vi "array -- bilinear regression 3D -- V2.vi"(7 "action":T3, 9 "fit map IN":map{T1, dbl}(c390), 11 "xywz IN":T2={"x"=[0.0, 0.0, 0.0, -1.0, -1.0, -1.0, 1.0, 1.0, 1.0], "y"=[-1.0, 0.0, 1.0, -1.0, 0.0, 1.0, -1.0, 0.0, 1.0], "z"=[1.0, 0.0, 1.0, 4.0, 1.0, 0.0, 0.0, 1.0, 4.0], "w"=[-1.0, 0.0, 1.0, -1.0, 0.0, 1.0, -1.0, 0.0, 1.0]}) -> (1 "fit map out":map{T1, dbl}(c390), 3 "xywz OUT":T2={"x"=[0.0, 0.0, 0.0, -1.0, -1.0, -1.0, 1.0, 1.0, 1.0], "y"=[-1.0, 0.0, 1.0, -1.0, 0.0, 1.0, -1.0, 0.0, 1.0], "z"=[1.0, 0.0, 1.0, 4.0, 1.0, 0.0, 0.0, 1.0, 4.0], "w"=[-1.0, 0.0, 1.0, -1.0, 0.0, 1.0, -1.0, 0.0, 1.0]})   [LabVIEW 2021]
uses:
  array -- fit control .ctl
  array -- bilinear regression 2D.ctl
  <vilib>/Analysis/baseanly.llb/Matrix Type of Inverse Matrix.ctl
  <vilib>/Analysis/baseanly.llb/Real A x B.vi
  <vilib>/Analysis/Matrix/Numeric/Conversions/Array To Matrix - RA2.vi
  <vilib>/Analysis/baseanly.llb/Real Inverse Matrix.vi
  <vilib>/Analysis/Matrix/Numeric/Conversions/Matrix To Array - RM.vi
  <vilib>/Analysis/NI_AALBase.lvlib
  <vilib>/Analysis/Matrix/NI_Matrix.lvlib
panel:
  out "w":dbl[](array[numeric])=[-1.0, 0.0, 1.0, -1.0, 0.0, 1.0, -1.0, 0.0, 1.0]
  out "y":dbl[](array[numeric])=[-1.0, 0.0, 1.0, -1.0, 0.0, 1.0, -1.0, 0.0, 1.0]
  out "fit  IN":dbl[](array[numeric])=[1.9, 2.6, 3.3, 1.0, 2.7, 3.9]
  out "fit OUT":dbl[](array[numeric])=[1.0, 1.0, 1.0, 0.0, 0.0, 0.0]
  out "z":dbl[](array[numeric])=[1.0, 0.0, 1.0, 4.0, 1.0, 0.0, 0.0, 1.0, 4.0]
  out "x":dbl[](array[numeric])=[0.0, 0.0, 0.0, -1.0, -1.0, -1.0, 1.0, 1.0, 1.0]
  # "s"
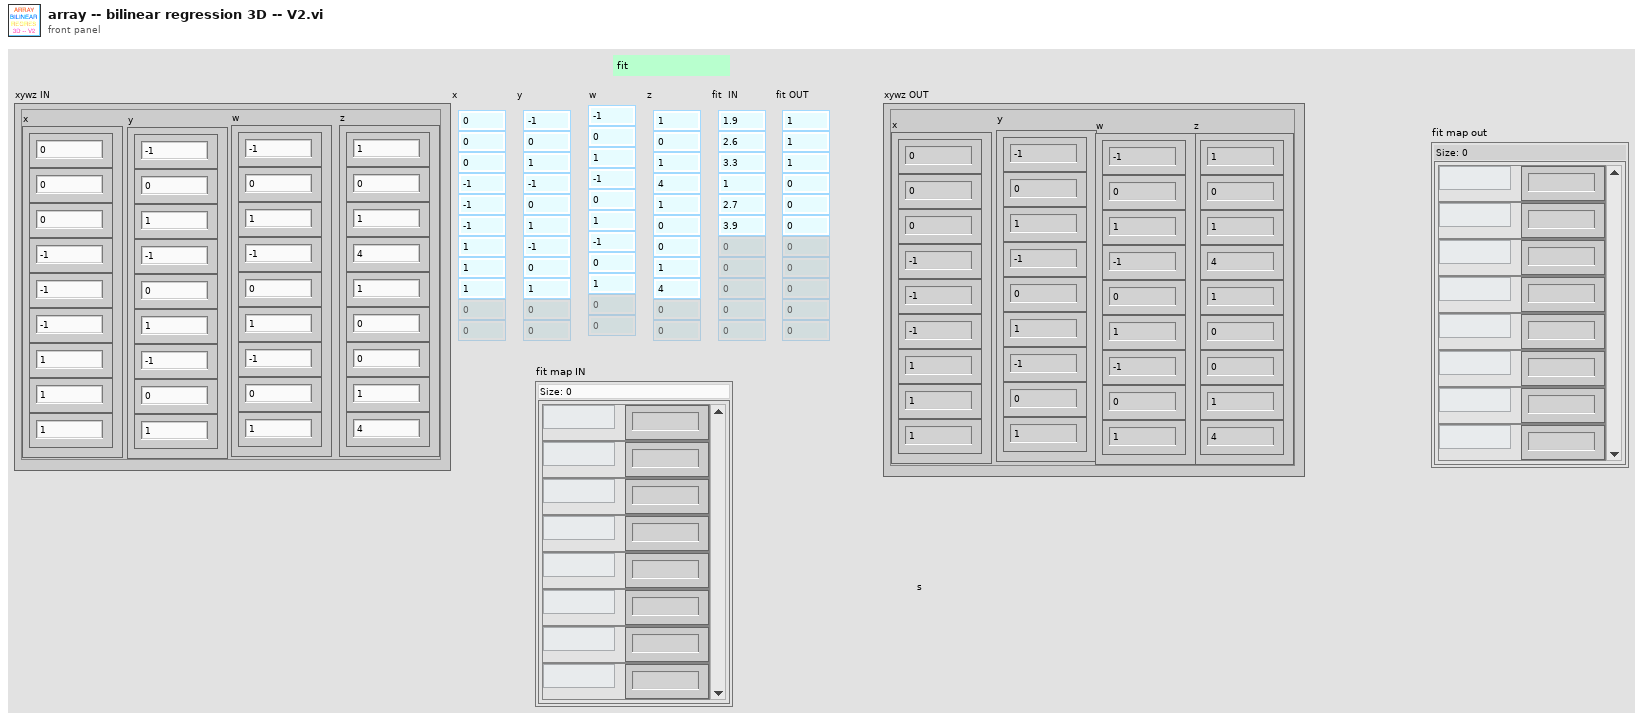
[diagram p1: front panel]
types:
  T1 = typedef "array -- bilinear regression 2D.ctl" = enum16{"1", "x", "y", "xx", "xy", "yy", "xxy", "xyy", "yyy", "xxx", "xxyy", "xyyy", "xxxy", "yyyy", "xxxx", "xxz", "xyz", "yyz", "xz", "yz", "z", "wwz", "ywz", "xwz", "xxxw", "xxyw", "xyyw", "yyyw", "xxww", "xyww", "yyww", "xwww", "ywww", "wwww", "ww", "xw", "yw", "w", "wz"}
  T2 = cluster{"x":dbl[], "y":dbl[], "z":dbl[], "w":dbl[]}
  T3 = typedef "array -- fit control .ctl" = enum16{"fit", "calc", "check", "init"}
  T4 = typedef "NI_AALBase.lvlib/Matrix Type of Inverse Matrix.ctl" = enum32{"General", "Positive Definite", "Lower Triangular", "Upper Triangular"}
  T5 = typedef "NI_Matrix.lvlib/RealMatrix.ctl" = dbl[][]
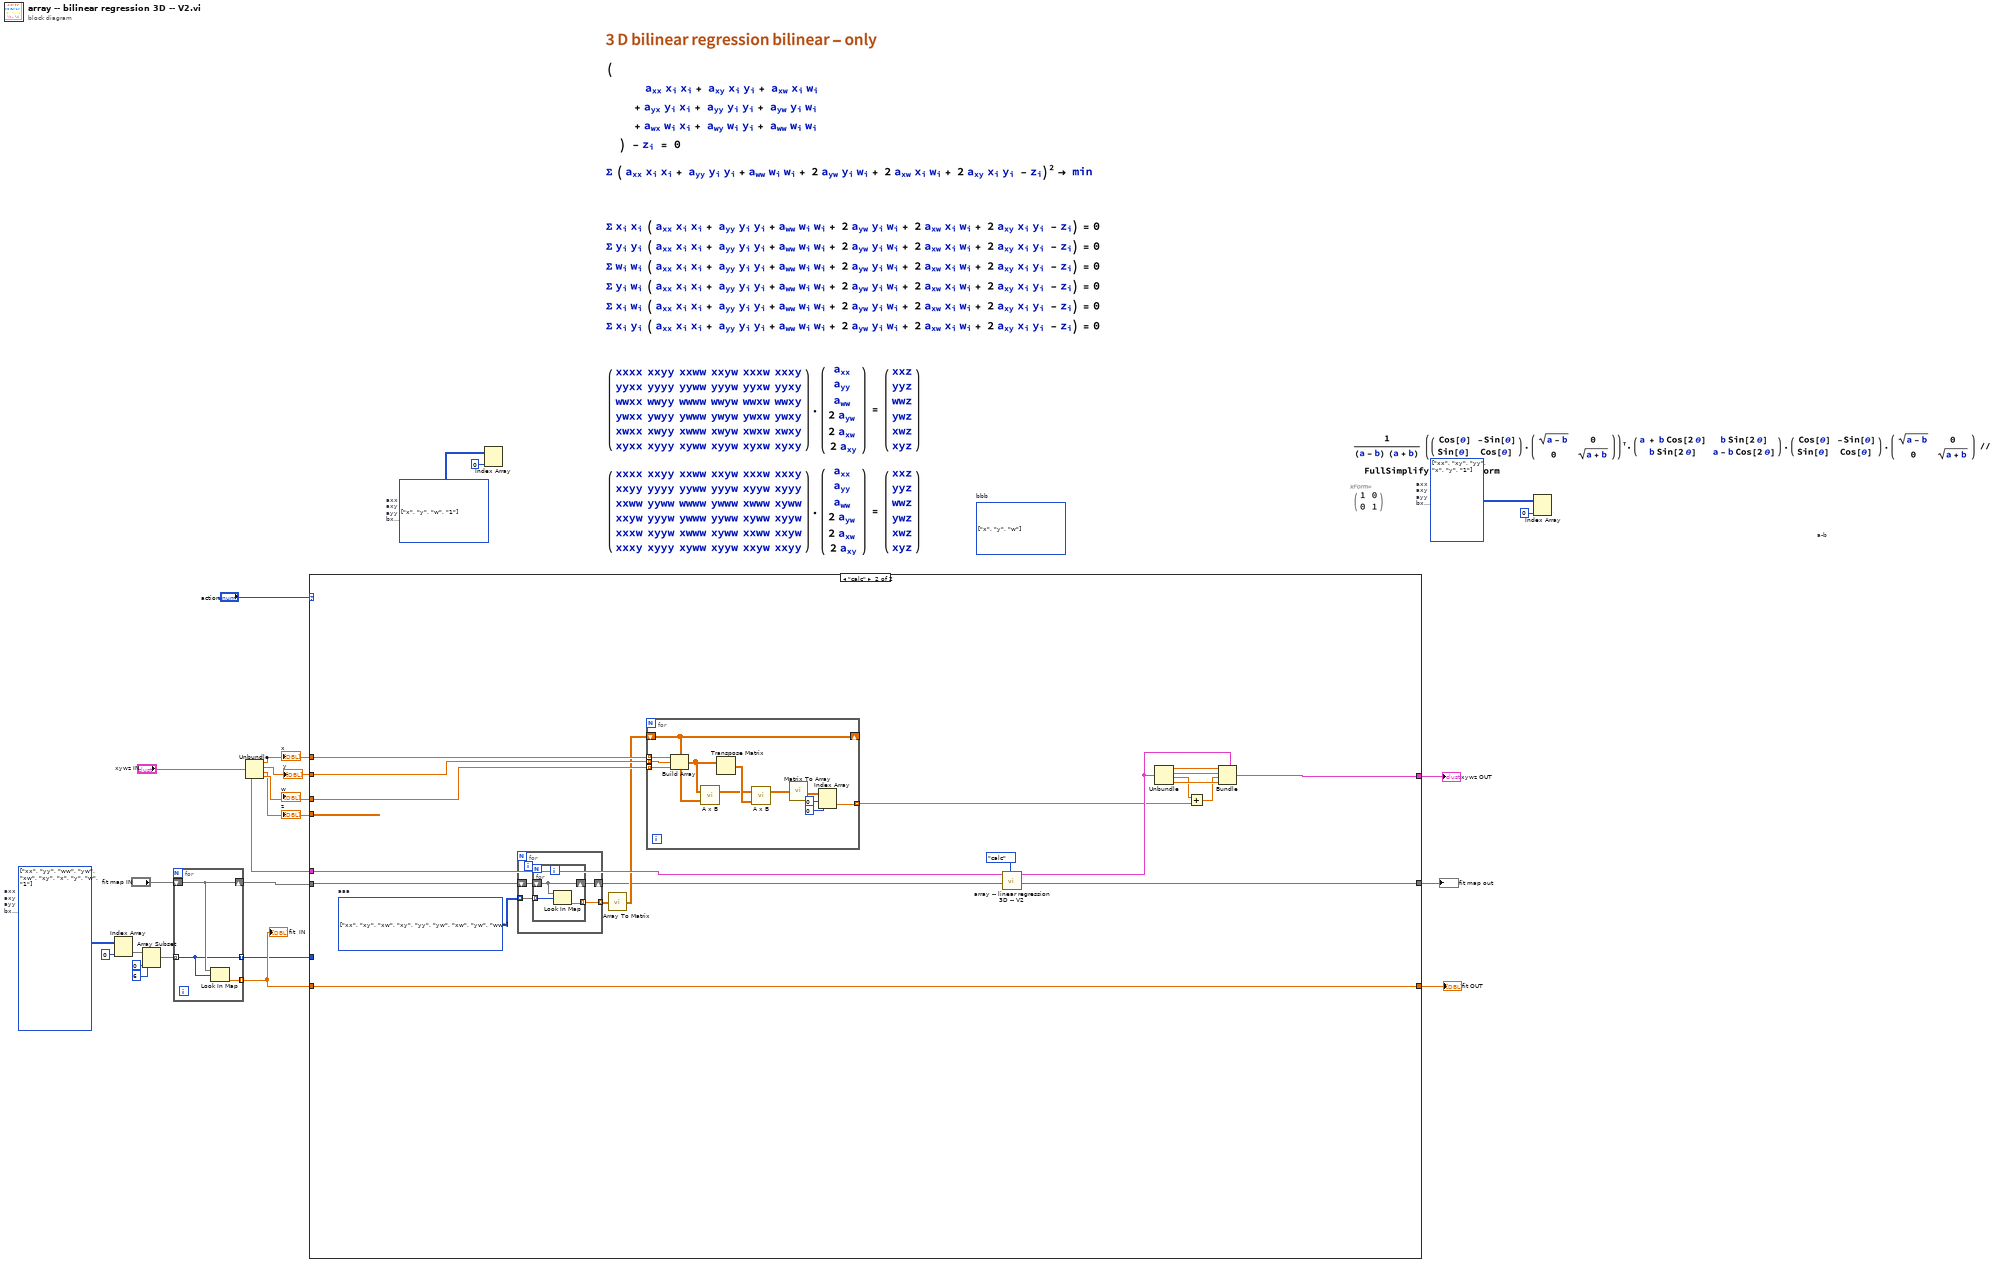
[diagram p0: block diagram]
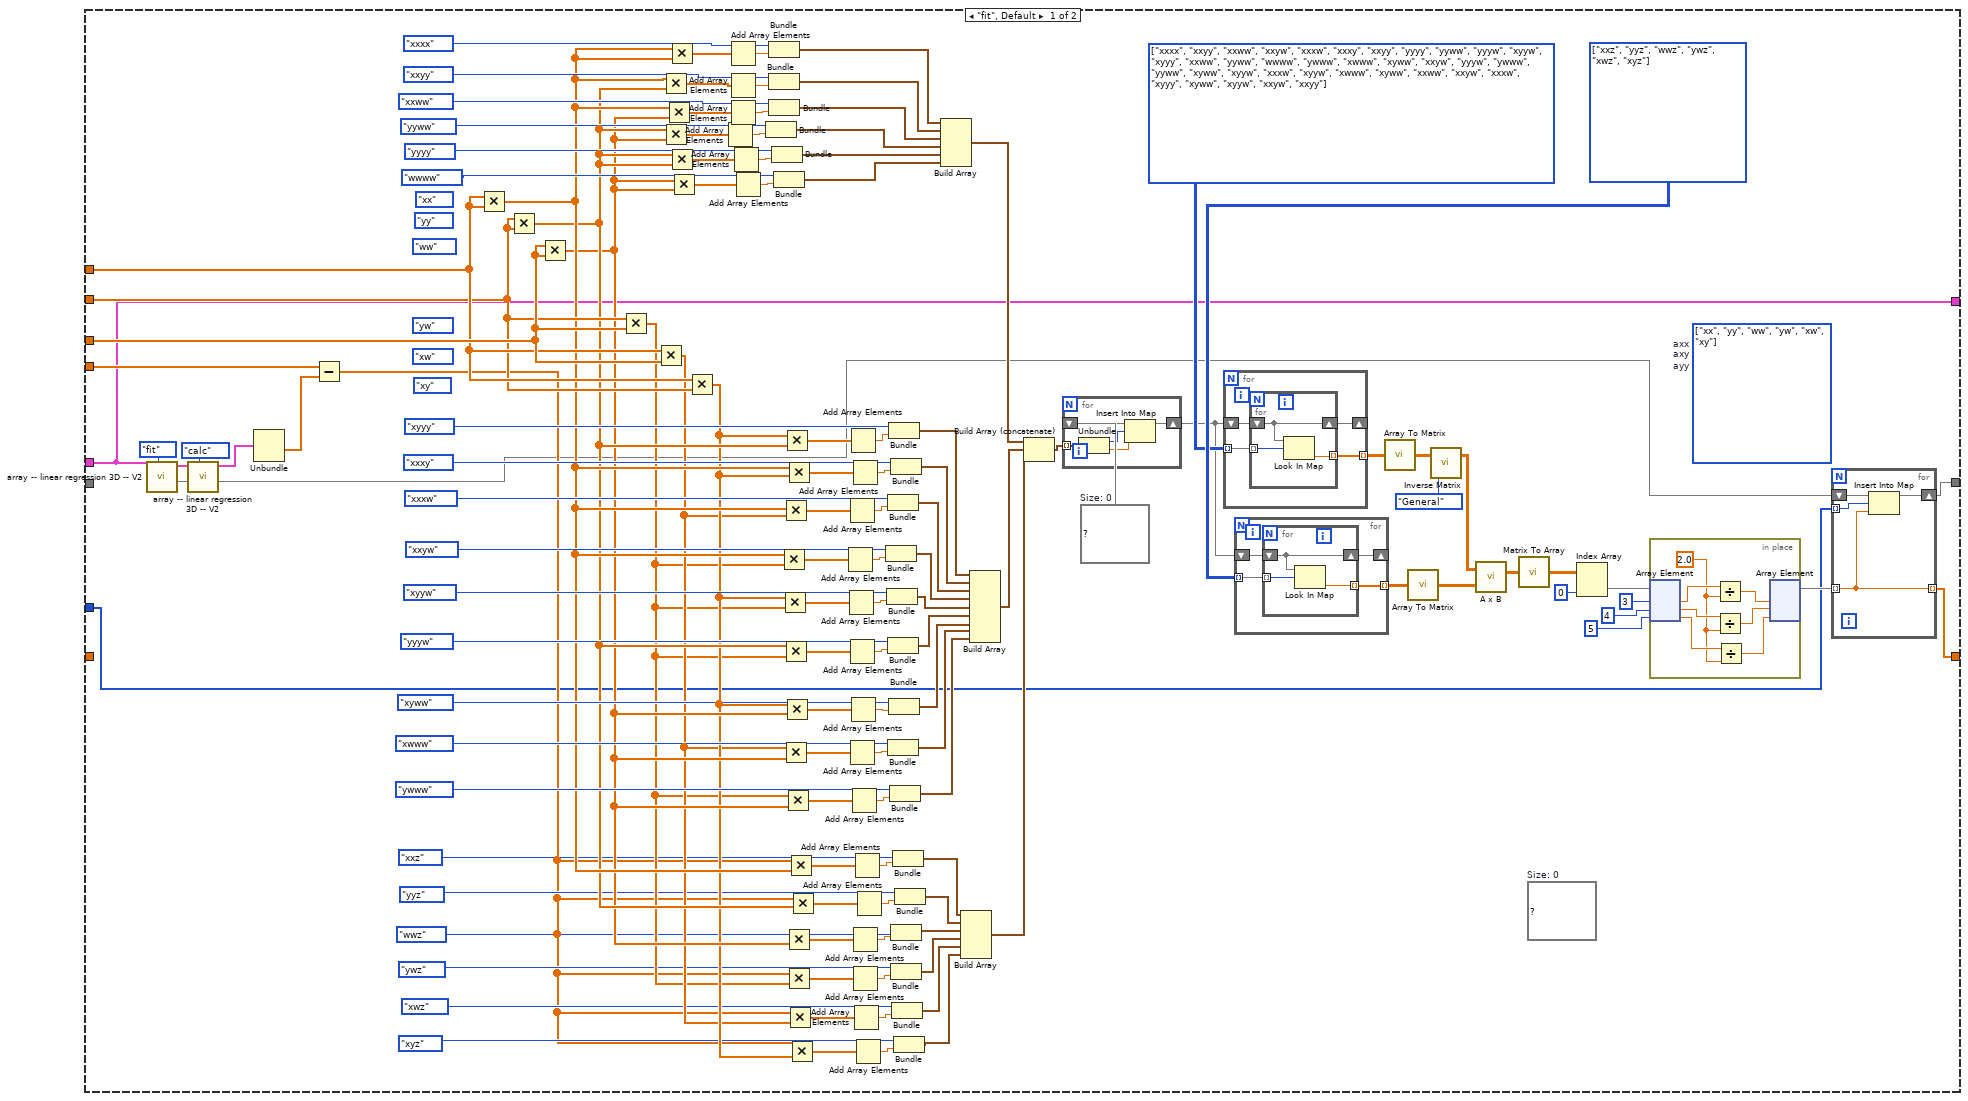
[diagram p2: hidden frame]
diagram:
  (unwired) T1[][] [[enum."x"], [enum."y"], [enum."w"]] items=["1", "x", "y", "xx", "xy", "yy", "xxy", "xyy", "yyy", "xxx", "xxyy", "xyyy", "xxxy", "yyyy", "xxxx", "xxz", "xyz", "yyz", "xz", "yz", "z", "wwz", "ywz", "xwz", "xxxw", "xxyw", "xyyw", "yyyw", "xxww", "xyww", "yyww", "xwww", "ywww", "wwww", "ww", "xw", "yw", "w", "wz"]  # bbb
  w15 = T1[][] [[enum."x"], [enum."y"], [enum."w"], [enum."1"]] items=["1", "x", "y", "xx", "xy", "yy", "xxy", "xyy", "yyy", "xxx", "xxyy", "xyyy", "xxxy", "yyyy", "xxxx", "xxz", "xyz", "yyz", "xz", "yz", "z", "wwz", "ywz", "xwz", "xxxw", "xxyw", "xyyw", "yyyw", "xxww", "xyww", "yyww", "xwww", "ywww", "wwww", "ww", "xw", "yw", "w", "wz"]  # axx axy ayy bx by c
  w17 = T1[][] [[enum."xx"], [enum."yy"], [enum."ww"], [enum."yw"], [enum."xw"], [enum."xy"], [enum."x"], [enum."y"], [enum."w"], [enum."1"]] items=["1", "x", "y", "xx", "xy", "yy", "xxy", "xyy", "yyy", "xxx", "xxyy", "xyyy", "xxxy", "yyyy", "xxxx", "xxz", "xyz", "yyz", "xz", "yz", "z", "wwz", "ywz", "xwz", "xxxw", "xxyw", "xyyw", "yyyw", "xxww", "xyww", "yyww", "xwww", "ywww", "wwww", "ww", "xw", "yw", "w", "wz"]  # axx axy ayy bx by c
  w19 = T1[][] [[enum."xx"], [enum."xy"], [enum."yy"], [enum."x"], [enum."y"], [enum."1"]] items=["1", "x", "y", "xx", "xy", "yy", "xxy", "xyy", "yyy", "xxx", "xxyy", "xyyy", "xxxy", "yyyy", "xxxx", "xxz", "xyz", "yyz", "xz", "yz", "z", "wwz", "ywz", "xwz", "xxxw", "xxyw", "xyyw", "yyyw", "xxww", "xyww", "yyww", "xwww", "ywww", "wwww", "ww", "xw", "yw", "w", "wz"]  # axx axy ayy bx by c
  # "a-b"
  n1 = Index Array(array=w17, index (col)=0 ("disabled index (col)")) -> (element=w12:T1[])  [unwired: 1 in]
  n2 = Array Subset(array=w12, index=0, length=6) -> (w3:T1[])
  n3 = for {
    shift-right: [w25] -> w2
    shift-left: "fit map IN" -> [w25]
    tunnel: w3 -> [w24] mode=indexing
    tunnel: [w26] -> w4 mode=indexing
    tunnel: [w24] -> w1 mode=indexing
    n4 = Look In Map(map=w25, key=w24) -> (value=w26:dbl)  [unwired: 1 in, 1 out]
  }
  "fit  IN" <- w4
  n5 = Unbundle("xywz IN") -> ("x"=w22:dbl[], "y"=w21:dbl[], "z"=w6:dbl[], "w"=w13:dbl[])
  "x" <- w22
  "z" <- w6
  "y" <- w21
  "w" <- w13
  n6 = case shown="\"calc\"" "action" {
    tunnel: w6 -> [w38 _]
    tunnel: w22 -> [w111 w200]
    tunnel: [w27 w187] -> w20
    tunnel: w21 -> [w110 w199]
    tunnel: w13 -> [w112 w198]
    tunnel: w2 -> [_ w188]
    tunnel: "xywz IN" -> [w31 w203]
    tunnel: [w31 w189] -> w9
    tunnel: [w40 w185] -> w8
    tunnel: w4 -> [_ w187]
    tunnel: w1 -> [w29 _]
    frame "fit", Default {
      (unwired) T1[][] [[enum."xx"], [enum."yy"], [enum."ww"], [enum."yw"], [enum."xw"], [enum."xy"]] items=["1", "x", "y", "xx", "xy", "yy", "xxy", "xyy", "yyy", "xxx", "xxyy", "xyyy", "xxxy", "yyyy", "xxxx", "xxz", "xyz", "yyz", "xz", "yz", "z", "wwz", "ywz", "xwz", "xxxw", "xxyw", "xyyw", "yyyw", "xxww", "xyww", "yyww", "xwww", "ywww", "wwww", "ww", "xw", "yw", "w", "wz"]  # axx axy ayy
      (unwired) map{T1, dbl} {}  # Size: 0
      w131 = T1[][] [[enum."xxz"], [enum."yyz"], [enum."wwz"], [enum."ywz"], [enum."xwz"], [enum."xyz"]] items=["1", "x", "y", "xx", "xy", "yy", "xxy", "xyy", "yyy", "xxx", "xxyy", "xyyy", "xxxy", "yyyy", "xxxx", "xxz", "xyz", "yyz", "xz", "yz", "z", "wwz", "ywz", "xwz", "xxxw", "xxyw", "xyyw", "yyyw", "xxww", "xyww", "yyww", "xwww", "ywww", "wwww", "ww", "xw", "yw", "w", "wz"]
      w130 = T1[][] [[enum."xxxx", enum."xxyy", enum."xxww", enum."xxyw", enum."xxxw", enum."xxxy"], [enum."xxyy", enum."yyyy", enum."yyww", enum."yyyw", enum."xyyw", enum."xyyy"], [enum."xxww", enum."yyww", enum."wwww", enum."ywww", enum."xwww", enum."xyww"], [enum."xxyw", enum."yyyw", enum."ywww", enum."yyww", enum."xyww", enum."xyyw"], [enum."xxxw", enum."xyyw", enum."xwww", enum."xyww", enum."xxww", enum."xxyw"], [enum."xxxw", enum."xyyy", enum."xyww", enum."xyyw", enum."xxyw", enum."xxyy"]] items=["1", "x", "y", "xx", "xy", "yy", "xxy", "xyy", "yyy", "xxx", "xxyy", "xyyy", "xxxy", "yyyy", "xxxx", "xxz", "xyz", "yyz", "xz", "yz", "z", "wwz", "ywz", "xwz", "xxxw", "xxyw", "xyyw", "yyyw", "xxww", "xyww", "yyww", "xwww", "ywww", "wwww", "ww", "xw", "yw", "w", "wz"]
      w133 = map{T1, dbl} {}  # Size: 0
      (unwired) array_--_bilinear_regression_2D."xy"
      (unwired) array_--_bilinear_regression_2D."xw"
      (unwired) array_--_bilinear_regression_2D."yw"
      (unwired) array_--_bilinear_regression_2D."ww"
      (unwired) array_--_bilinear_regression_2D."yy"
      (unwired) array_--_bilinear_regression_2D."xx"
      n7 = call "array -- linear regression 3D -- V2.vi"("action"=array_--_fit_control_."fit", "xyzw IN"=w31) -> ("fit map out"=w36:map{T1, dbl}, "xyz OUT"=w35:T2)  [unwired: 8 in]
      n8 = call "array -- linear regression 3D -- V2.vi"("action"=array_--_fit_control_."calc", "fit map IN"=w36, "xyzw IN"=w35) -> ("fit map out"=w32:map{T1, dbl}, "xyz OUT"=w37:T2)  [unwired: 7 in]
      n9 = Unbundle(w37) -> ("z"=w30:dbl[])  [unwired: 3 out]
      n10 = Subtract(x=w38, y=w30) -> (x-y=w39:dbl[])
      n11 = Multiply(x=w111, y=w111) -> (x*y=w55:dbl[])
      n12 = Multiply(x=w110, y=w110) -> (x*y=w54:dbl[])
      n13 = Multiply(x=w112, y=w112) -> (x*y=w53:dbl[])
      n14 = Multiply(x=w110, y=w112) -> (x*y=w50:dbl[])
      n15 = Multiply(x=w111, y=w112) -> (x*y=w51:dbl[])
      n16 = Multiply(x=w55, y=w54) -> (x*y=w126:dbl[])
      n17 = Multiply(x=w54, y=w53) -> (x*y=w123:dbl[])
      n18 = Multiply(x=w55, y=w53) -> (x*y=w125:dbl[])
      n19 = Multiply(x=w55, y=w55) -> (x*y=w149:dbl[])
      n20 = Multiply(x=w54, y=w54) -> (x*y=w121:dbl[])
      n21 = Multiply(x=w53, y=w53) -> (x*y=w119:dbl[])
      n22 = Multiply(x=w111, y=w110) -> (x*y=w52:dbl[])
      n23 = Add Array Elements(numeric array=w123) -> (sum=w124:dbl)
      n24 = Add Array Elements(numeric array=w149) -> (sum=w148:dbl)
      n25 = Add Array Elements(numeric array=w126) -> (sum=w146:dbl)
      n26 = Add Array Elements(numeric array=w125) -> (sum=w143:dbl)
      n27 = Add Array Elements(numeric array=w121) -> (sum=w122:dbl)
      n28 = Add Array Elements(numeric array=w119) -> (sum=w120:dbl)
      n29 = Bundle(array_--_bilinear_regression_2D."yyww", "Numeric"=w124) -> (w118:cluster{T1, "Numeric":dbl})  [unwired: 1 in]
      n30 = Bundle(array_--_bilinear_regression_2D."xxxx", "Numeric"=w148) -> (w127:cluster{T1, "Numeric":dbl})  [unwired: 1 in]
      n31 = Bundle(array_--_bilinear_regression_2D."xxyy", "Numeric"=w146) -> (w128:cluster{T1, "Numeric":dbl})  [unwired: 1 in]
      n32 = Bundle(array_--_bilinear_regression_2D."xxww", "Numeric"=w143) -> (w129:cluster{T1, "Numeric":dbl})  [unwired: 1 in]
      n33 = Bundle(array_--_bilinear_regression_2D."yyyy", "Numeric"=w122) -> (w114:cluster{T1, "Numeric":dbl})  [unwired: 1 in]
      n34 = Bundle(array_--_bilinear_regression_2D."wwww", "Numeric"=w120) -> (w113:cluster{T1, "Numeric":dbl})  [unwired: 1 in]
      n35 = Multiply(x=w55, y=w50) -> (x*y=w104:dbl[])
      n36 = Multiply(x=w52, y=w50) -> (x*y=w102:dbl[])
      n37 = Multiply(x=w55, y=w51) -> (x*y=w106:dbl[])
      n38 = Multiply(x=w54, y=w50) -> (x*y=w100:dbl[])
      n39 = Multiply(x=w51, y=w53) -> (x*y=w96:dbl[])
      n40 = Multiply(x=w52, y=w54) -> (x*y=w154:dbl[])
      n41 = Multiply(x=w52, y=w53) -> (x*y=w98:dbl[])
      n42 = Multiply(x=w50, y=w53) -> (x*y=w94:dbl[])
      n43 = Multiply(x=w55, y=w52) -> (x*y=w108:dbl[])
      n44 = Multiply(x=w39, y=w53) -> (x*y=w66:dbl[])
      n45 = Multiply(x=w39, y=w50) -> (x*y=w68:dbl[])
      n46 = Multiply(x=w39, y=w51) -> (x*y=w70:dbl[])
      n47 = Multiply(x=w39, y=w55) -> (x*y=w62:dbl[])
      n48 = Multiply(x=w39, y=w52) -> (x*y=w72:dbl[])
      n49 = Multiply(x=w39, y=w54) -> (x*y=w64:dbl[])
      n50 = Add Array Elements(numeric array=w104) -> (sum=w105:dbl)
      n51 = Add Array Elements(numeric array=w102) -> (sum=w103:dbl)
      n52 = Add Array Elements(numeric array=w106) -> (sum=w107:dbl)
      n53 = Add Array Elements(numeric array=w100) -> (sum=w101:dbl)
      n54 = Add Array Elements(numeric array=w96) -> (sum=w97:dbl)
      n55 = Add Array Elements(numeric array=w154) -> (sum=w141:dbl)
      n56 = Add Array Elements(numeric array=w98) -> (sum=w99:dbl)
      n57 = Add Array Elements(numeric array=w94) -> (sum=w95:dbl)
      n58 = Add Array Elements(numeric array=w108) -> (sum=w109:dbl)
      n59 = Add Array Elements(numeric array=w66) -> (sum=w67:dbl)
      n60 = Add Array Elements(numeric array=w68) -> (sum=w69:dbl)
      n61 = Add Array Elements(numeric array=w70) -> (sum=w71:dbl)
      n62 = Add Array Elements(numeric array=w62) -> (sum=w63:dbl)
      n63 = Add Array Elements(numeric array=w72) -> (sum=w73:dbl)
      n64 = Add Array Elements(numeric array=w64) -> (sum=w65:dbl)
      n65 = Bundle(array_--_bilinear_regression_2D."xxyw", "Numeric"=w105) -> (w79:cluster{T1, "Numeric":dbl})  [unwired: 1 in]
      n66 = Bundle(array_--_bilinear_regression_2D."xyyw", "Numeric"=w103) -> (w78:cluster{T1, "Numeric":dbl})  [unwired: 1 in]
      n67 = Bundle(array_--_bilinear_regression_2D."xxxw", "Numeric"=w107) -> (w80:cluster{T1, "Numeric":dbl})  [unwired: 1 in]
      n68 = Bundle(array_--_bilinear_regression_2D."yyyw", "Numeric"=w101) -> (w77:cluster{T1, "Numeric":dbl})  [unwired: 1 in]
      n69 = Bundle(array_--_bilinear_regression_2D."xwww", "Numeric"=w97) -> (w75:cluster{T1, "Numeric":dbl})  [unwired: 1 in]
      n70 = Bundle(array_--_bilinear_regression_2D."xyyy", "Numeric"=w141) -> (w82:cluster{T1, "Numeric":dbl})  [unwired: 1 in]
      n71 = Bundle(array_--_bilinear_regression_2D."xyww", "Numeric"=w99) -> (w76:cluster{T1, "Numeric":dbl})  [unwired: 1 in]
      n72 = Bundle(array_--_bilinear_regression_2D."ywww", "Numeric"=w95) -> (w74:cluster{T1, "Numeric":dbl})  [unwired: 1 in]
      n73 = Bundle(array_--_bilinear_regression_2D."xxxy", "Numeric"=w109) -> (w81:cluster{T1, "Numeric":dbl})  [unwired: 1 in]
      n74 = Bundle(array_--_bilinear_regression_2D."wwz", "Numeric"=w67) -> (w59:cluster{T1, "Numeric":dbl})  [unwired: 1 in]
      n75 = Bundle(array_--_bilinear_regression_2D."ywz", "Numeric"=w69) -> (w58:cluster{T1, "Numeric":dbl})  [unwired: 1 in]
      n76 = Bundle(array_--_bilinear_regression_2D."xwz", "Numeric"=w71) -> (w57:cluster{T1, "Numeric":dbl})  [unwired: 1 in]
      n77 = Bundle(array_--_bilinear_regression_2D."xxz", "Numeric"=w63) -> (w61:cluster{T1, "Numeric":dbl})  [unwired: 1 in]
      n78 = Bundle(array_--_bilinear_regression_2D."xyz", "Numeric"=w73) -> (w56:cluster{T1, "Numeric":dbl})  [unwired: 1 in]
      n79 = Bundle(array_--_bilinear_regression_2D."yyz", "Numeric"=w65) -> (w60:cluster{T1, "Numeric":dbl})  [unwired: 1 in]
      n80 = Build Array(w127, w128, w129, w118, w114, w113) -> (w84:cluster{T1, "Numeric":dbl}[])
      n81 = Build Array(w61, w60, w59, w58, w57, w56) -> (w43:cluster{T1, "Numeric":dbl}[])
      n82 = Build Array(w82, w81, w80, w79, w78, w77, w76, w75, w74) -> (w83:cluster{T1, "Numeric":dbl}[])
      n83 = Build Array (concatenate)(w84, w83, w43) -> (w85:cluster{T1, "Numeric":dbl}[])
      n84 = for {
        tunnel: w85 -> [w175] mode=indexing
        shift-right: [w176] -> w28
        shift-left: w133 -> [w177]
        n85 = Unbundle(w175) -> (w174:T1, "Numeric"=w173:dbl)
        n86 = Insert Into Map(map in=w177, key=w174, value=w173) -> (map out=w176:map{T1, dbl})  [unwired: 2 out]
      }
      n87 = for {
        tunnel: w130 -> [w181] mode=indexing
        shift-right: [w179] -> _
        shift-left: w28 -> [w180]
        tunnel: [w178] -> w139 mode=indexing
        n88 = for {
          tunnel: w181 -> [w183] mode=indexing
          shift-right: [w184] -> w179
          shift-left: w180 -> [w184]
          tunnel: [w182] -> w178 mode=indexing
          n89 = Look In Map(map=w184, key=w183) -> (value=w182:dbl)  [unwired: 1 in, 1 out]
        }
      }
      n90 = for {
        shift-right: [w168] -> _
        shift-left: w28 -> [w169]
        tunnel: w131 -> [w167] mode=indexing
        tunnel: [w166] -> w138 mode=indexing
        n91 = for {
          shift-right: [w172] -> w168
          shift-left: w169 -> [w172]
          tunnel: w167 -> [w171] mode=indexing
          tunnel: [w170] -> w166 mode=indexing
          n92 = Look In Map(map=w172, key=w171) -> (value=w170:dbl)  [unwired: 1 in, 1 out]
        }
      }
      n93 = call-poly <vilib>:"Array To Matrix.vi"("Real 2D Array"=w139) -> ("Real Matrix"=w134:T5)
      n94 = call-poly <vilib>:"Array To Matrix.vi"("Real 2D Array"=w138) -> ("Real Matrix"=w137:T5)
      n95 = call-poly <vilib>:"Inverse Matrix.vi"("matrix type"=Matrix_Type_of_Inverse_Matrix."General", "Input Matrix"=w134) -> ("Inverse Matrix"=w153:T5)  [unwired: 1 out]
      n96 = call-poly <vilib>:"A x B.vi"("B"=w137, "A"=w153) -> ("A x B"=w152:T5)  [unwired: 1 out]
      n97 = call-poly <vilib>:"Matrix To Array.vi"("Real Matrix"=w152) -> ("Real 2D Array"=w151:dbl[][])
      n98 = Index Array(array=w151, index (col)=0 ("disabled index (col)")) -> (element=w136:dbl[])  [unwired: 1 in]
      n99 = in-place {
        w159 = 2.0 ("y")
        n100 = in-place-array #1(w136, 3, 4, 5) -> (w165:dbl, w163:dbl, w161:dbl)
        n101 = Divide(x=w165, y=w159) -> (x/y=w164:dbl)
        n102 = Divide(x=w163, y=w159) -> (x/y=w162:dbl)
        n103 = Divide(x=w161, y=w159) -> (x/y=w160:dbl)
        n104 = in-place-array #1(w164, w162, w160) -> (w132:dbl[])  [unwired: 3 out]
      }
      n105 = for {
        shift-right: [w157] -> w40
        shift-left: w32 -> [w158]
        tunnel: w29 -> [w156] mode=indexing
        tunnel: w132 -> [w155] mode=indexing
        tunnel: [w155] -> w27 mode=indexing
        n106 = Insert Into Map(map in=w158, key=w156, value=w155) -> (map out=w157:map{T1, dbl})  [unwired: 2 out]
      }
    }
    frame "calc" {
      w201 = T1[][] [[enum."xx", enum."xy", enum."xw"], [enum."xy", enum."yy", enum."yw"], [enum."xw", enum."yw", enum."ww"]] items=["1", "x", "y", "xx", "xy", "yy", "xxy", "xyy", "yyy", "xxx", "xxyy", "xyyy", "xxxy", "yyyy", "xxxx", "xxz", "xyz", "yyz", "xz", "yz", "z", "wwz", "ywz", "xwz", "xxxw", "xxyw", "xyyw", "yyyw", "xxww", "xyww", "yyww", "xwww", "ywww", "wwww", "ww", "xw", "yw", "w", "wz"]  # aaa
      n107 = for {
        tunnel: w201 -> [w220] mode=indexing
        shift-right: [w218] -> w186
        shift-left: w188 -> [w219]
        tunnel: [w217] -> w202 mode=indexing
        n108 = for {
          tunnel: w220 -> [w222] mode=indexing
          shift-right: [w223] -> w218
          shift-left: w219 -> [w223]
          tunnel: [w221] -> w217 mode=indexing
          n109 = Look In Map(map=w223, key=w222) -> (value=w221:dbl)  [unwired: 1 in, 1 out]
        }
      }
      n110 = call-poly <vilib>:"Array To Matrix.vi"("Real 2D Array"=w202) -> ("Real Matrix"=w197:T5)
      n111 = for {
        tunnel: w200 -> [w215] mode=indexing
        tunnel: w199 -> [w214] mode=indexing
        tunnel: w198 -> [w213] mode=indexing
        shift-right: [w212] -> _
        shift-left: w197 -> [w212]
        tunnel: [w205] -> w190 mode=indexing
        n112 = Build Array(w215, w214, w213) -> (w211:T5)
        n113 = call-poly <vilib>:"A x B.vi"("B"=w212, "A"=w211) -> ("A x B"=w209:T5)  [unwired: 1 out]
        n114 = Transpose Matrix(1:w211) -> (0:w210:T5)
        n115 = call-poly <vilib>:"A x B.vi"("B"=w210, "A"=w209) -> ("A x B"=w216:T5)  [unwired: 1 out]
        n116 = call-poly <vilib>:"Matrix To Array.vi"("Real Matrix"=w216) -> ("Real 2D Array"=w208:dbl[][])
        n117 = Index Array(array=w208, index (row)=0, index (col)=0 ("disabled index (col)")) -> (element=w205:dbl)
      }
      n118 = call "array -- linear regression 3D -- V2.vi"("action"=array_--_fit_control_."calc", "fit map IN"=w186, "xyzw IN"=w203) -> ("fit map out"=w185:map{T1, dbl}, "xyz OUT"=w196:T2)  [unwired: 7 in]
      n119 = Unbundle(w196) -> ("x"=w195:dbl[], "y"=w194:dbl[], "z"=w192:dbl[], "w"=w193:dbl[])
      n120 = Add(x=w192, y=w190) -> (x+y=w191:dbl[])
      n121 = Bundle(cluster=w196, "x"=w195, "y"=w194, "z"=w191, "w"=w193) -> (w189:T2)
    }
  }
  "fit OUT" <- w20
  "fit map out" <- w8
  "xywz OUT" <- w9
  n122 = Index Array(array=w15, index (col)=0 ("disabled index (col)")) -> ()  [unwired: 1 in, 1 out]
  n123 = Index Array(array=w19, index (col)=0 ("disabled index (col)")) -> ()  [unwired: 1 in, 1 out]
